vi "Align two Waveforms (single shot).vi"(4 "interpolation":bool=TRUE, 5 "exported interval":u16(ring) items=["common", "global"], 6 "FIR filter specifications":T1={"alias rejection (dB)"=120.0, "normalized bandwidth"=0.4536} {"normalized bandwidth" format="%.4f"; "alias rejection (dB)" format="%.2f"}, 7 "open interval? (T)":bool=TRUE, 8 "error in (no error)":errorcluster, 9 "interpolation mode":u16(ring)=1 items=["coerce", "linear", "spline", "FIR filter"], 10 "waveform B in":waveform(dbl), 11 "waveform A in":waveform(dbl)) -> (0 "error out":errorcluster, 2 "waveform B out":waveform(dbl), 3 "waveform A out":waveform(dbl))   [LabVIEW 2020, in "NI_MAPro.lvlib"]
doc: "Performs element-wise alignment of two waveforms and returns the aligned waveforms. The data types you wire to the waveform inputs determine the polymorphic instance to use."
uses:
  NI_MAPro.lvlib
panel:
  # "open"
  # "closed"
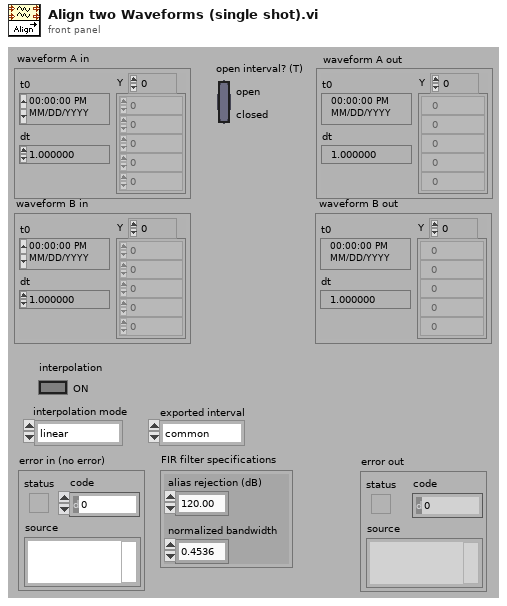
[diagram p1: front panel]
types:
  T1 = cluster{"alias rejection (dB)":dbl, "normalized bandwidth":dbl}
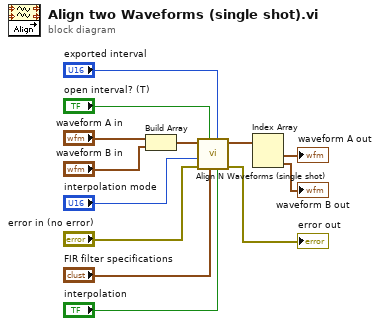
[diagram p0: block diagram]
diagram:
  n1 = Build Array("waveform A in", "waveform B in") -> (w13:waveform(dbl)[])
  n2 = call "Align N Waveforms (single shot).vi"("interpolation"="interpolation", "exported interval"="exported interval", "FIR filter specifications"="FIR filter specifications", "open interval? (T)"="open interval? (T)", "error in (no error)"="error in (no error)", "interpolation mode"="interpolation mode", "waveforms in"=w13) -> ("error out"=→"error out":errorcluster, "aligned waveforms out"=w12:waveform(dbl)[])  [unwired: 3 in]
  n3 = Index Array(array=w12) -> (element #1=→"waveform A out":waveform(dbl), element #2=→"waveform B out":waveform(dbl))  [unwired: 2 in]
